vi "TestNotLoggingAnyData.vi"() -> ()   [LabVIEW 2018]
uses:
  feGEM DataPacker.lvlib
panel:
  in  "stop":bool
  out "error out":errorcluster
  in  "MIDAS Server":string="my_midas_server.domain"
  in  "MIDAS Sever Port":u16=12345
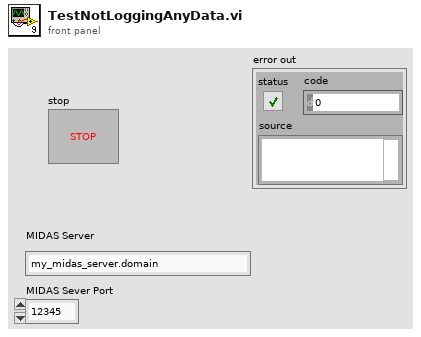
[diagram p1: front panel]
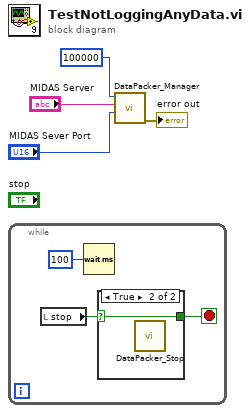
[diagram p0: block diagram]
diagram:
  n1 = while {
    stop <- w6 stop-if-true
    n2 = local read "stop"() -> (w5:bool)
    n3 = Wait (ms)(milliseconds to wait=u32 100) -> ()  [unwired: 1 out]
    n4 = case shown="True" w5 {
      selector: w5 -> [w8 w9]
      tunnel: [w8 w9] -> w6
      frame False {
      }
      frame True {
        n5 = call "DataPacker_Stop.vi"() -> ()  [unwired: 12 in]
      }
    }
  }
  n6 = call "DataPacker_Manager.vi"("MIDAS Sever Port"="MIDAS Sever Port", "MIDAS Server"="MIDAS Server", "Override Max Event size (Data rate bytes/s). Use MIDAS Default = 0"=u32 100000 ("Override Max Event size (Data rate kb/s). Use MIDAS Default = 0")) -> ("error out"=→"error out":errorcluster)  [unwired: 8 in]
